vi "SetGXMLCfgStrain.vi"(8 "error in (no error)":errorcluster, 10 "StrainChanCfg":T1, 11 "Strain in":refnum<class "Strain.lvclass">) -> (0 "error out":errorcluster, 3 "Strain out":refnum<class "Strain.lvclass">)   [LabVIEW 2012, in "Measurement Channels.lvlib" / "Strain.lvclass"]
uses:
  Strain.lvclass
  StrainProps_TD.ctl
  Strain.lvclass/Strain.ctl
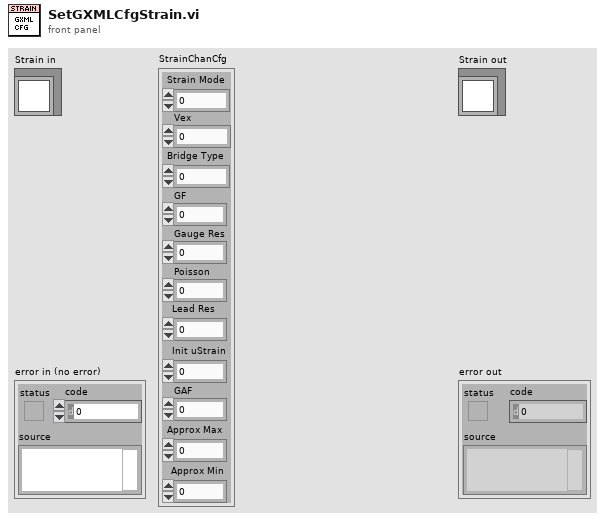
[diagram p1: front panel]
types:
  T1 = typedef "Measurement Channels.lvlib/Strain.lvclass/StrainProps_TD.ctl" = cluster{"Strain Mode":u16, "Vex":dbl, "Bridge Type":u16, "GF":dbl, "Gauge Res":i32, "Poisson":dbl, "Lead Res":dbl, "Init uStrain":dbl, "GAF":dbl, "Approx Max":dbl, "Approx Min":dbl}
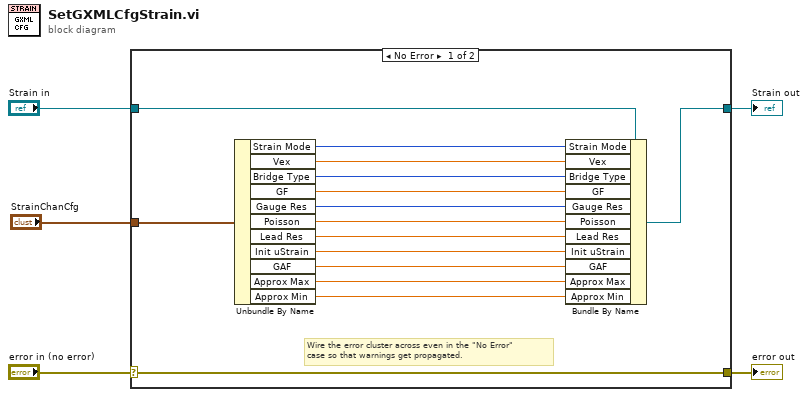
[diagram p0: block diagram]
diagram:
  n1 = case shown="No Error" "error in (no error)" {
    selector: "error in (no error)" -> [w20 w22]
    tunnel: [w20 w22] -> w4
    tunnel: [w6 w21] -> w2
    tunnel: "Strain in" -> [w7 w21]
    tunnel: "StrainChanCfg" -> [w8 _]
    frame No Error {
      # "Wire the error cluster across even in the \"No Error\"\ncase so that warnings get propagated."
      n2 = Unbundle By Name(w8) -> ("Strain Mode"=w19:u16, "Vex"=w18:dbl, "Bridge Type"=w17:u16, "GF"=w16:dbl, "Gauge Res"=w15:i32, "Poisson"=w14:dbl, "Lead Res"=w13:dbl, "Init uStrain"=w12:dbl, "GAF"=w11:dbl, "Approx Max"=w10:dbl, "Approx Min"=w9:dbl)
      n3 = Bundle By Name(cluster=w7, "Strain Mode"=w19, "Vex"=w18, "Bridge Type"=w17, "GF"=w16, "Gauge Res"=w15, "Poisson"=w14, "Lead Res"=w13, "Init uStrain"=w12, "GAF"=w11, "Approx Max"=w10, "Approx Min"=w9) -> (w6:refnum<class "Strain.lvclass">)
    }
    frame Error {
    }
  }
  "error out" <- w4
  "Strain out" <- w2
